vi "B_3.vi"() -> ()   [LabVIEW 2020]
uses:
  <vilib>/numeric/Random Number (Range) U64.vi
  <vilib>/numeric/sub_Random U32.vi
panel:
  in  "Beginning":bool
  in  "stop":bool
  out "Table":u64[](array[numeric])
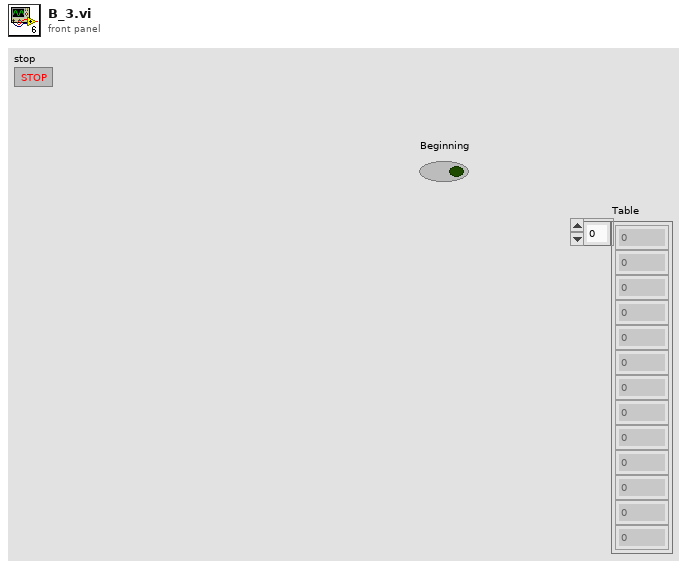
[diagram p1: front panel]
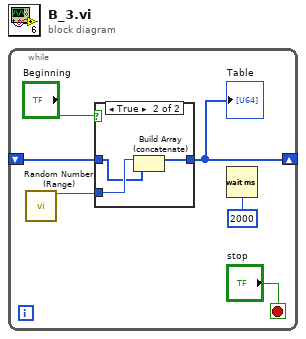
[diagram p0: block diagram]
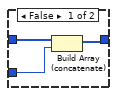
[diagram p2: hidden frame]
diagram:
  n1 = while {
    shift-right: [w3] -> _
    shift-left: _ -> [w4]
    stop <- "stop" stop-if-true
    n2 = call-poly <vilib>:"Random Number (Range).vi"() -> ("number"=w5:u64)  [unwired: 11 in]
    n3 = case shown="True" "Beginning" {
      tunnel: w5 -> [w8 w11]
      tunnel: w4 -> [w9 w10]
      tunnel: [w7 w12] -> w3
      frame False {
        n4 = Build Array (concatenate)(w9, w8) -> (w7:u64[])
      }
      frame True {
        n5 = Build Array (concatenate)(w11, w10) -> (w12:u64[])
      }
    }
    "Table" <- w3
    n6 = Wait (ms)(milliseconds to wait=u32 2000) -> ()  [unwired: 1 out]
  }
